vi "value to ring (FrameStartMode).vi"(11 "value":string) -> (3 "FrameStartMode":i32(ring)=1 items=["FDX_TX_FRAME_START_IFG", "FDX_TX_FRAME_START_PGWT", "FDX_TX_FRAME_START_TRG", "FDX_TX_FRAME_START_TRG_D"])   [LabVIEW 2020, in "AIM ARINC 664 Import.lvlib"]
uses:
  AIM ARINC 664 Import.lvlib
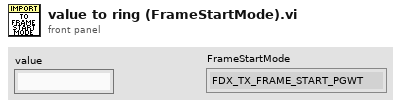
[diagram p1: front panel]
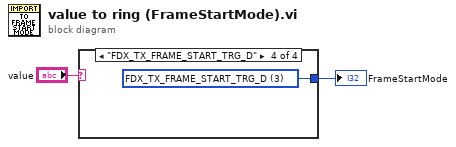
[diagram p0: block diagram]
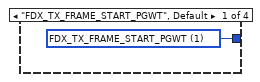
[diagram p2: hidden frame]
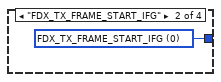
[diagram p3: hidden frame]
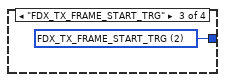
[diagram p4: hidden frame]
diagram:
  n1 = case shown="\"FDX_TX_FRAME_START_TRG_D\"" "value" {
    tunnel: [w3 w4 w5 w6] -> w1
    frame "FDX_TX_FRAME_START_PGWT", Default {
      w3 = 1 items=["FDX_TX_FRAME_START_IFG", "FDX_TX_FRAME_START_PGWT", "FDX_TX_FRAME_START_TRG", "FDX_TX_FRAME_START_TRG_D"] ("FrameStartMode")
    }
    frame "FDX_TX_FRAME_START_IFG" {
      w4 = 0 items=["FDX_TX_FRAME_START_IFG", "FDX_TX_FRAME_START_PGWT", "FDX_TX_FRAME_START_TRG", "FDX_TX_FRAME_START_TRG_D"] ("FrameStartMode")
    }
    frame "FDX_TX_FRAME_START_TRG" {
      w5 = 2 items=["FDX_TX_FRAME_START_IFG", "FDX_TX_FRAME_START_PGWT", "FDX_TX_FRAME_START_TRG", "FDX_TX_FRAME_START_TRG_D"] ("FrameStartMode")
    }
    frame "FDX_TX_FRAME_START_TRG_D" {
      w6 = 3 items=["FDX_TX_FRAME_START_IFG", "FDX_TX_FRAME_START_PGWT", "FDX_TX_FRAME_START_TRG", "FDX_TX_FRAME_START_TRG_D"] ("FrameStartMode")
    }
  }
  "FrameStartMode" <- w1
